vi "lockin.TestLauncher.vi"() -> ()   [LabVIEW 2016, in "lockin.lvclass"]
uses:
  lockin.lvclass
  <vilib>/JKI/JKI SMO/SMO/Typedefs/SMOState --Enum.ctl
  Typedefs/output_config.ctl
  Typedefs/lockin_config.ctl
  C:/Program Files (x86)/National Instruments/LabVIEW 2016/vi.lib/JKI/JKI SMO/SMO/SMO.lvclass
  <vilib>/JKI/JKI SMO/SMO/SMO.lvclass
panel:
  in  "Channel":dbl
  out "Y/R":dbl format="%#_6p"
  out "X/R":dbl format="%#_6p"
  out "Waveform Chart 2":waveform(dbl)[](graph)
  out "Waveform Chart":waveform(dbl)[](graph)
  in  "Display":enum16{"X and Y", "R and Theta"}(ring)=enum."R and Theta"
  out "REF":waveform(dbl)[](graph)
  in  "lockin config":T1
  in  "output config":T2=[{"A (V)"=1.0, "DC (V)"=0.0, "f (Hz)"=1.0, "phi (deg)"=0.0, "signal type"=enum."Sine Wave"}, {"A (V)"=2.0, "DC (V)"=0.0, "f (Hz)"=2.0, "phi (deg)"=0.0, "signal type"=enum."Sine Wave"}, {"A (V)"=3.0, "DC (V)"=0.0, "f (Hz)"=3.0, "phi (deg)"=0.0, "signal type"=enum."Sine Wave"}, {"A (V)"=4.0, "DC (V)"=0.0, "f (Hz)"=4.0, "phi (deg)"=0.0, "signal type"=enum."Sine Wave"}, {"A (V)"=5.0, "DC (V)"=0.0, "f (Hz)"=5.0, "phi (deg)"=0.0, "signal type"=enum."Sine Wave"}, {"A (V)"=6.0, "DC (V)"=0.0, "f (Hz)"=6.0, "phi (deg)"=0.0, "signal type"=enum."Sine Wave"}, {"A (V)"=7.0, "DC (V)"=0.0, "f (Hz)"=7.0, "phi (deg)"=0.0, "signal type"=enum."Sine Wave"}]
  out "Write":T3(graph)
  out "Read":waveform(dbl)[](graph)
  out "SMO State":T4
  out "error out":errorcluster
  in  "Stop":bool
  # "use network streams to pass data between different computers?\nOr ZeroMQ?\nhave lockin running on different (or same) computers\none is AO/AI\nThe other is lockin DSP"
  # "LOCKIN: Basic SMO Test Launcher"
  # "For instructions on how to use the JKI State Machine Objects, examples and video tutorials, visit:\nhttp://jki.net/state-machine-objects/\n\nJKI State Machine Objects™\nhttp://jki.net/state-machine-objects/\nCopyright (C) 2005-2015, JKI <info@jki.net>\nALL RIGHTS RESERVED"
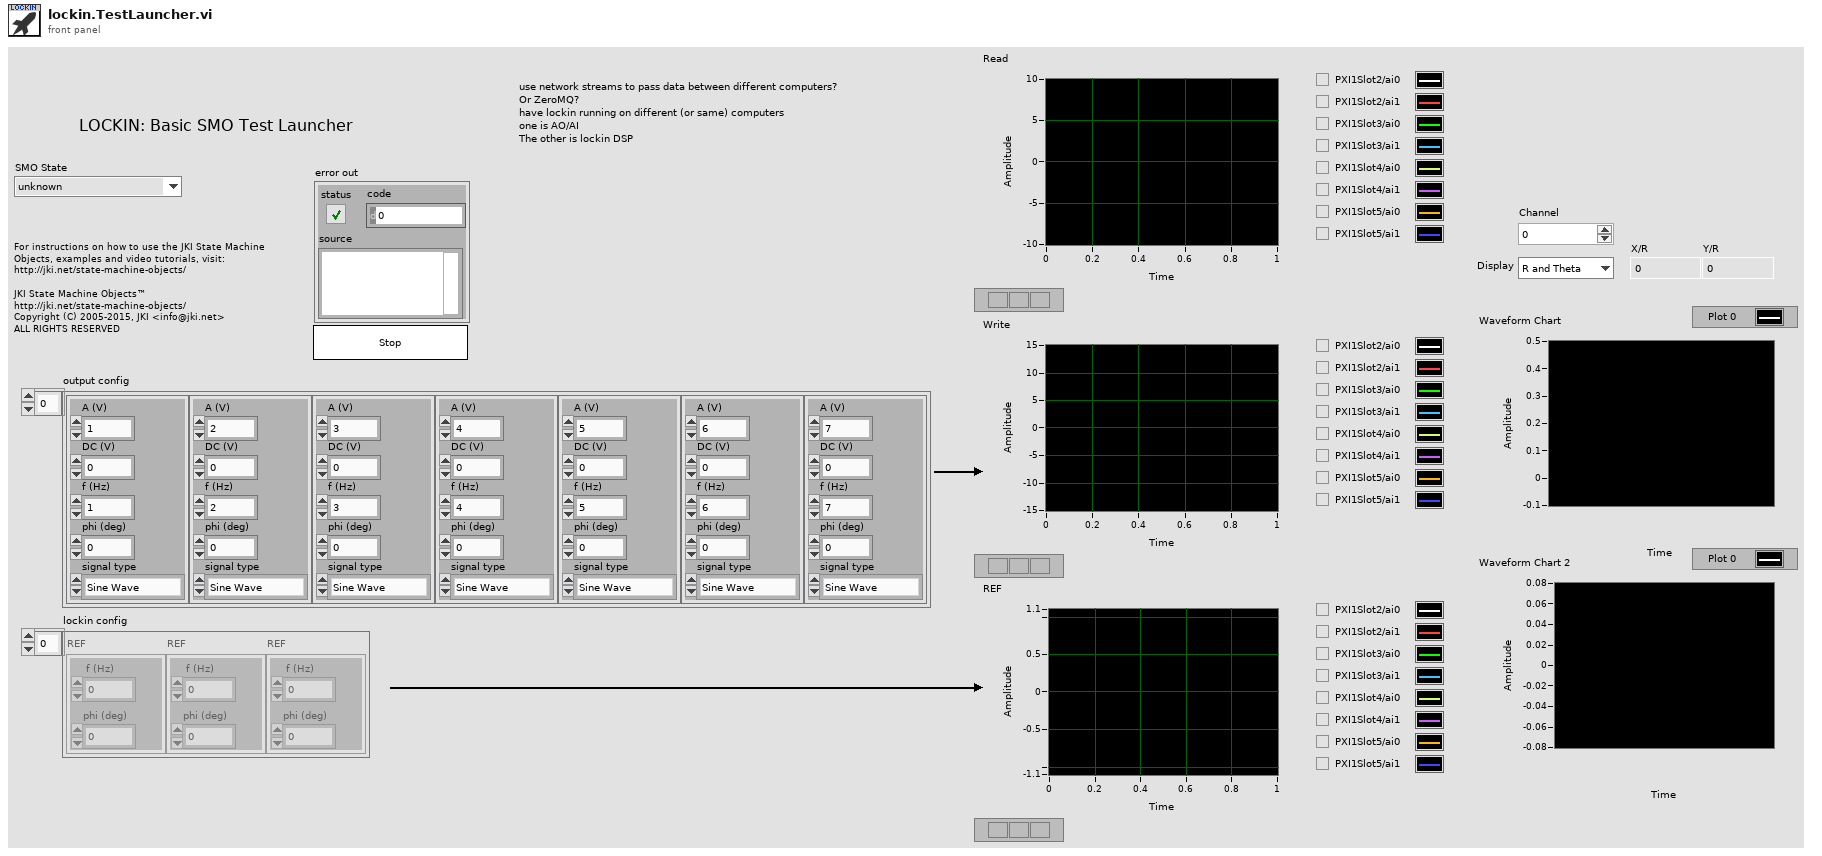
[diagram p1: front panel]
types:
  T1 = typedef "lockin.lvclass/lockin_config.ctl" = cluster{" f (Hz)":dbl, "phi (deg)":dbl}[]
  T2 = typedef "lockin.lvclass/output_config.ctl" = cluster{"A (V)":dbl, "DC (V)":dbl, "f (Hz)":dbl, "phi (deg)":dbl, "signal type":enum16{"Sine Wave", "Triangle Wave", "Square Wave", "Sawtooth Wave"}}[]
  T3 = typedef "lockin.lvclass/PublicEvents--lockin.Write.ctl" = waveform(dbl)[]
  T4 = typedef "SMO.lvclass/SMOState --Enum.ctl" = enum16{"unknown", "Created", "Started", "Stopped"}
  T5 = typedef "SMO.lvclass/Public Events.ctl" = cluster{"Error":refnum<user-event>, "State":refnum<user-event>, "Reserve State":refnum<user-event>}
  T6 = typedef "lockin.lvclass/PublicEvents--Cluster.ctl" = cluster{"read":refnum<user-event>, "Write":refnum<user-event>, "lockin_REF_waveform":refnum<user-event>, "lockin_results":refnum<user-event>}
  T7 = cluster{"Event Registration Refnum":refnum<event-registration>}
  T8 = typedef "lockin.lvclass/PublicEvents--lockin.read.ctl" = waveform(dbl)[]
  T9 = typedef "lockin.lvclass/PublicEvents--lockin.lockin_REF_waveform.ctl" = waveform(dbl)[]
  T10 = typedef "lockin.lvclass/PublicEvents--lockin.lockin_results.ctl" = dbl[][]
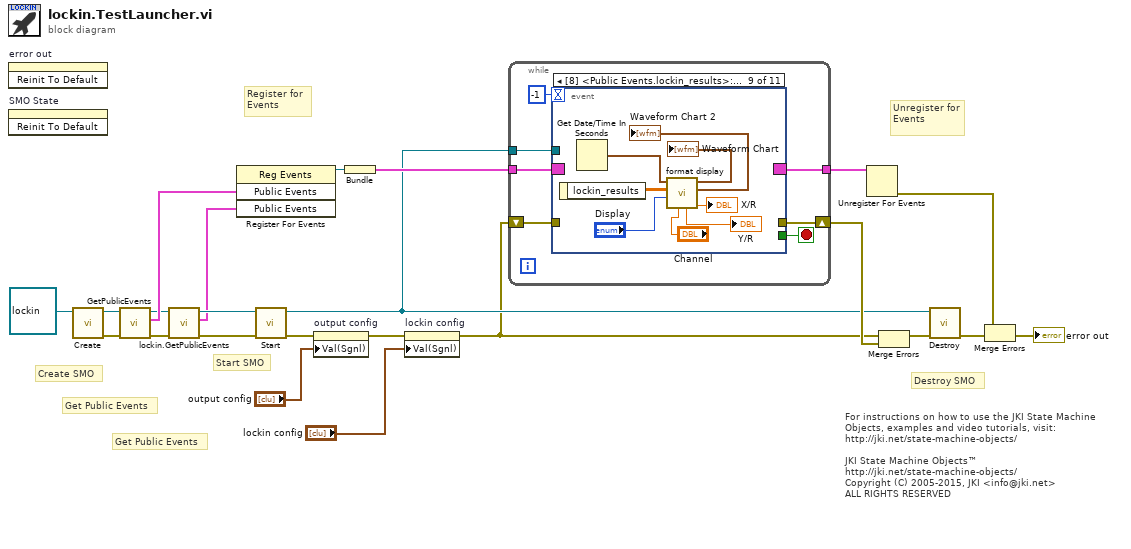
[diagram p0: block diagram]
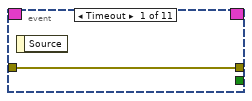
[diagram p2: hidden frame]
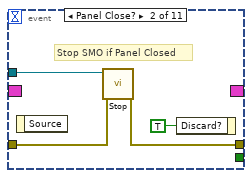
[diagram p3: hidden frame]
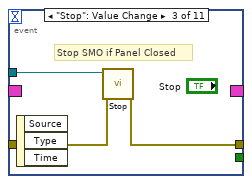
[diagram p4: hidden frame]
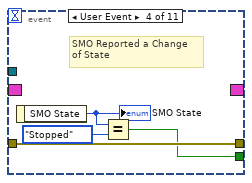
[diagram p5: hidden frame]
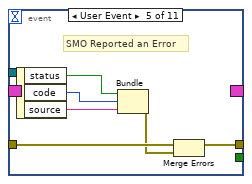
[diagram p6: hidden frame]
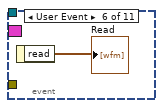
[diagram p7: hidden frame]
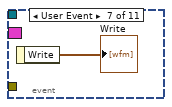
[diagram p8: hidden frame]
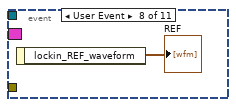
[diagram p9: hidden frame]
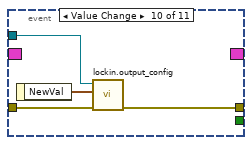
[diagram p10: hidden frame]
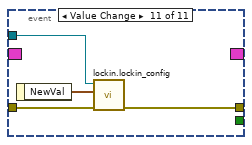
[diagram p11: hidden frame]
diagram:
  # "Get Public Events"
  # "For instructions on how to use the JKI State Machine Objects, examples and video tutorials, visit:\nhttp://jki.net/state-machine-objects/\n\nJKI State Machine Objects™\nhttp://jki.net/state-machine-objects/\nCopyright (C) 2005-2015, JKI <info@jki.net>\nALL RIGHTS RESERVED"
  # "Get Public Events"
  # "Start SMO"
  # "Destroy SMO"
  # "Create SMO"
  # "Unregister for Events"
  # "Register for Events"
  n1 = invoke on="error out" class="Clust (strict)" method="Reinit To Default"() -> ()  [unwired: 3 in, 3 out]
  n2 = invoke on="SMO State" class="Enum (strict)" method="Reinit To Default"() -> ()  [unwired: 3 in, 3 out]
  n3 = call <vilib>:"Create.vi"("SMO"=refnum<class "lockin.lvclass"> refnum ("SMO.Template.lvclass")) -> ("error out"=w14:errorcluster, "SMO out"=w15:refnum<class "lockin.lvclass">)  [unwired: 8 in, 1 out]
  n4 = call <vilib>:"GetPublicEvents.vi"("error in (no error)"=w14, "SMO"=w15) -> ("error out"=w10:errorcluster, "Public Events"=w13:T5, "SMO out"=w11:refnum<class "lockin.lvclass">)  [unwired: 7 in]
  n5 = call "lockin.GetPublicEvents.vi"("error in (no error)"=w10, "lockin"=w11) -> ("error out"=w8:errorcluster, "Public Events"=w4:T6, "lockin out"=w9:refnum<class "lockin.lvclass">)  [unwired: 7 in]
  n6 = register-events(w13, w4) -> (reference out=w12:refnum<event-registration>)  [unwired: 2 in, 1 out]
  n7 = call <vilib>:"Start.vi"("error in (no error)"=w8, "SMO"=w9) -> ("error out"=w6:errorcluster, "SMO out"=w7:refnum<class "lockin.lvclass">)  [unwired: 8 in]
  n8 = property on="output config" class="Arr (strict)"(error in=w6, "Val(Sgnl)"="output config") -> (error out=w3:errorcluster)  [unwired: 1 in, 1 out]
  n9 = Bundle("Event Registration Refnum"=w12) -> (w22:T7)  [unwired: 1 in]
  n10 = property on="lockin config" class="Arr (strict)"(error in=w3, "Val(Sgnl)"="lockin config") -> (error out=w2:errorcluster)  [unwired: 1 in, 1 out]
  n11 = while {
    shift-right: [w29] -> w21
    shift-left: w2 -> [w28]
    tunnel: w22 -> [w27]
    tunnel: [w26] -> w23
    tunnel: w7 -> [w25]
    stop <- w30 stop-if-true
    n12 = event shown="[8] <Public Events.lockin_results>: User Event" {
      selector: w27 -> [_ _ _ _ _ _ _ _ _ _ _]
      dyn-events: [_ _ _ _ _ _ _ _ _ _ _] -> w26
      timeout: -1 -> [_ _ _ _ _ _ _ _ _ _ _]
      tunnel: [_ _ _ w39 _ _ _ _ _ _ _] -> w30
      tunnel: w25 -> [_ w35 w38 _ _ _ _ _ _ w61 w66]
      tunnel: [w31 w34 w37 w42 w46 _ _ _ _ w62 w64] -> w29
      tunnel: w28 -> [w31 w33 w36 w42 w44 _ _ _ _ w63 w65]
      event Timeout {
        n13 = event-data() -> ()  [unwired: 1 in, 1 out]
      }
      event Panel Close? {
        # "Stop SMO if Panel Closed"
        n14 = event-data() -> ()  [unwired: 1 in, 1 out]
        n15 = call <vilib>:"Stop.vi"("error in (no error)"=w33, "SMO"=w35) -> ("error out"=w34:errorcluster)  [unwired: 8 in, 1 out]
        n16 = event-data("Discard?"=TRUE ("OK")) -> ()  [unwired: 1 in, 1 out]
      }
      event "Stop": Value Change {
        # "Stop SMO if Panel Closed"
        n17 = event-data() -> ()  [unwired: 1 in, 3 out]
        n18 = call <vilib>:"Stop.vi"("error in (no error)"=w36, "SMO"=w38) -> ("error out"=w37:errorcluster)  [unwired: 8 in, 1 out]
      }
      event User Event {
        # "SMO Reported a Change\nof State"
        n19 = event-data() -> ("SMO State"=w41:T4)  [unwired: 1 in]
        "SMO State" <- w41
        n20 = Equal?(x=w41, y=SMOState_--Enum."Stopped") -> (x = y?=w39:bool)
      }
      event User Event {
        # "SMO Reported an Error"
        n21 = event-data() -> ("status"=w45:bool, "code"=w48:i32, "source"=w47:string)  [unwired: 1 in]
        n22 = Bundle("status"=w45, "code"=w48, "source"=w47) -> (w43:errorcluster)  [unwired: 1 in]
        n23 = Merge Errors(w44, w43) -> (w46:errorcluster)
      }
      event User Event {
        n24 = event-data() -> ("read"=→"Read":T8)  [unwired: 1 in]
      }
      event User Event {
        n25 = event-data() -> ("Write"=→"Write":T3)  [unwired: 1 in]
      }
      event User Event {
        n26 = event-data() -> ("lockin_REF_waveform"=→"REF":T9)  [unwired: 1 in]
      }
      event User Event {
        n27 = event-data() -> ("lockin_results"=w59:T10)  [unwired: 1 in]
        n28 = Get Date/Time In Seconds() -> (seconds since 1Jan1904=w53:timestamp)
        n29 = call "format display.vi"("Channel"="Channel", "Display"="Display", "Results (X,Y,R,Theta)"=w59, "t0"=w53) -> ("X/R"=→"X/R":dbl, "Y/Theta Array"=→"Waveform Chart 2":waveform(dbl)[], "X/R Array"=→"Waveform Chart":waveform(dbl)[], "Y/R"=→"Y/R":dbl)  [unwired: 3 in, 1 out]
      }
      event Value Change {
        n30 = event-data() -> ("NewVal"=w60:T2)  [unwired: 1 in]
        n31 = call "lockin.output_config.vi"("error in (no error)"=w63, "output_config"=w60, "lockin"=w61) -> ("error out"=w62:errorcluster)  [unwired: 7 in, 1 out]
      }
      event Value Change {
        n32 = event-data() -> ("NewVal"=w67:T1)  [unwired: 1 in]
        n33 = call "lockin.lockin_config.vi"("error in (no error)"=w65, "lockin_config"=w67, "lockin"=w66) -> ("error out"=w64:errorcluster)  [unwired: 7 in, 1 out]
      }
    }
  }
  n34 = Unregister For Events(event registration refnum=w23) -> (error out=w20:errorcluster)  [unwired: 1 in]
  n35 = Merge Errors(w2, w21) -> (w16:errorcluster)
  n36 = call <vilib>:"Destroy.vi"("error in (no error)"=w16, "SMO"=w7) -> ("error out"=w18:errorcluster)  [unwired: 9 in]
  n37 = Merge Errors(w20, w18) -> (→"error out":errorcluster)
